vi "CreateDescriptionNode.vi"(8 "Error In":errorcluster, 10 "Pattern":T1, 11 "DOM Document":refnum<k20>) -> (0 "Error out":errorcluster, 3 "Description Node":refnum<k20>)   [LabVIEW 2012, in "Virtual-PGA.lvlib"]
uses:
  Virtual-PGA.lvlib
  Public/Controls/Pattern.ctl
  Public/Controls/Input.ctl
  <resource>/objmgr/DOMUserDefRef.rc
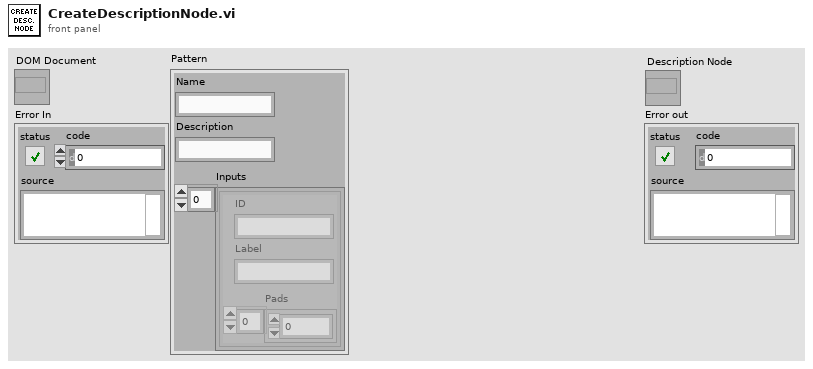
[diagram p1: front panel]
types:
  T1 = typedef "Virtual-PGA.lvlib/Pattern.ctl" = cluster{"Name":string, "Description":string, "Inputs":T2[]}
  T2 = typedef "Virtual-PGA.lvlib/Input.ctl" = cluster{"ID":string, "Label":string, "Pads":u32[]}
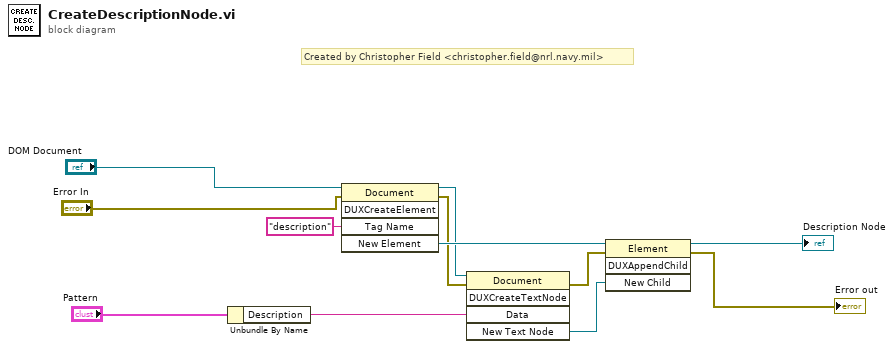
[diagram p0: block diagram]
diagram:
  # "Created by Christopher Field <christopher.field@nrl.navy.mil>"
  n1 = Unbundle By Name("Pattern") -> ("Description"=w1:string)
  n2 = invoke class="Document" method="DUXCreateElement"(reference="DOM Document", error in="Error In", "Tag Name"="description") -> (reference out=w5:refnum<k20>, error out=w4:errorcluster, "New Element"=w6:refnum<k20>)  [unwired: 2 in, 2 out]
  n3 = invoke class="Document" method="DUXCreateTextNode"(reference=w5, error in=w4, "Data"=w1) -> (error out=w3:errorcluster, "New Text Node"=w2:refnum<k20>)  [unwired: 2 in, 3 out]
  n4 = invoke class="Element" method="DUXAppendChild"(reference=w6, error in=w3, "New Child"=w2) -> (reference out=→"Description Node":refnum<k20>, error out=→"Error out":errorcluster)  [unwired: 1 in, 2 out]
